vi "Add DIO card.vi"(8 "error in (no error)":errorcluster, 11 "Node Ptr":u64 format="%.0x") -> (0 "error out":errorcluster)   [LabVIEW 2014, in "SLSC configuration System Explorer.lvlib"]
uses:
  SLSC configuration System Explorer.lvlib
  Shared/Constants.vi
  Shared/SLSC configuration Shared.lvlib
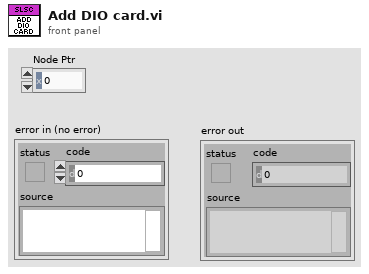
[diagram p1: front panel]
types:
  T1 = typedef "SLSC configuration Shared.lvlib/Card Position.ctl" = cluster{"Rack #":u8, "Slot #":T2}
  T2 = typedef "SLSC configuration Shared.lvlib/Slot #.ctl" = u8
  T3 = typedef "Custom Device API.lvlib/Custom Device Item Ref.ctl" = u64
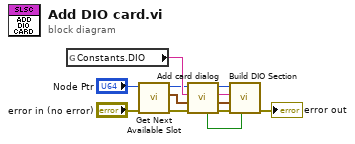
[diagram p0: block diagram]
diagram:
  n1 = global read "Constants.vi" "Constants.DIO"() -> (w8:string)
  n2 = call "Get Next Available Slot.vi"("error in (no error)"="error in (no error)", "Device Ref in"="Node Ptr") -> ("error out"=w5:errorcluster, "Next Open Slot"=w4:T1, "Device Ref out"=w2:T3)  [unwired: 7 in]
  n3 = call "Add card dialog.vi"("error in (no error)"=w5, "Card Position"=w4, "Card Type in"=w8, "Node Ptr"=w2) -> ("error out"=w12:errorcluster, "Card Position out"=w9:T1, "Name out"=w11:string, "Node Ptr out"=w10:u64, "Cancelled?"=w1:bool)  [unwired: 3 in]
  n4 = call "Build DIO Section.vi"("Cancelled?"=w1, "error in (no error)"=w12, "Card Position in"=w9, "Name in"=w11, "Node Ptr in"=w10) -> ("error out"=→"error out":errorcluster)  [unwired: 6 in]
